vi "Table verify colomn.vi"(0 "PDF Report":T21(xcontrol), 5 "numColumns":i32, 9 "columnWidth":sgl[](array[numeric]), 11 "error in (no error)":errorcluster, 12 "Pages dimensions":T1={"Start at page"=-1, "Orientation"=enum."Portrait", "widht"=612.0, "height"=792.0, "Margin left"=72.0, "Margin right"=72.0, "Margin top"=72.0, "Margin bottom"=72.0}) -> (4 "PDF Report duplicate":T21(xcontrol), 6 "numColumns duplicate":i32, 10 "columnWidth (points)":sgl[](array[numeric]), 15 "error out":errorcluster)   [LabVIEW 2013]
doc: "Version 1.0\nDeveloped by Jean-Marc Simard\nCopyright © 2010, Exaprom Inc.\nAll rights reserved.\nLicense: BSD\n\nWith iTextSharp 4.1.6 (http://itextsharp.sourceforge.net)\nunder Mozilla Public License Version 1.1\n(http://www.mozilla.org/MPL/MPL-1.1.html)"
uses:
  Controls/PDF Report Xcontrol/PDF Report.xctl
  Controls/Page dimensions.ctl
  Controls/Page Orientation.ctl
  Controls/Unit.ctl
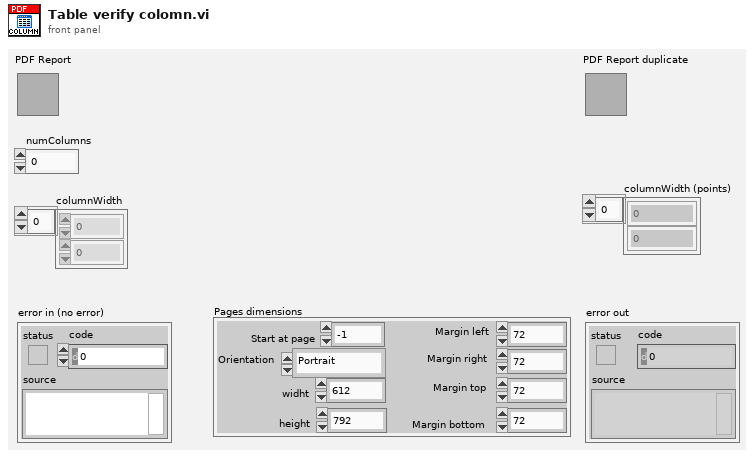
[diagram p1: front panel]
types:
  T1 = typedef "Page dimensions.ctl" = cluster{"Start at page":i32, "Orientation":T2, "widht":sgl, "height":sgl, "Margin left":sgl, "Margin right":sgl, "Margin top":sgl, "Margin bottom":sgl}
  T2 = typedef "Page Orientation.ctl" = enum16{"Portrait", "Landscape"}
  T3 = typedef "Font cluster.ctl" = cluster{"Name":string, "Size":T4, "Color":T5, "Style":cluster{"Bold":bool, "Italic":bool, "Underline":bool, "Strikeout":bool}}
  T4 = typedef "Font size.ctl" = sgl
  T5 = typedef "Font color.ctl" = u32
  T6 = typedef "Unit.ctl" = enum16{"inch", "mm"}
  T7 = typedef "Paragraphe cluster.ctl" = cluster{" Aligment":T8, "Line spacing":T9}
  T8 = typedef "Texte alignement.ctl" = enum16{"Select", "CENTER", "JUSTIFY", "LEFT", "RIGHT"}
  T9 = typedef "Line spacing.ctl" = enum16{"Select", "1.0", "1.5", "2.0"}
  T10 = typedef "Image or Table Caption.ctl" = cluster{"Caption":string, "Separator":string, "Position":enum16{"Above", "Below"}}
  T11 = typedef "Header Footer [ ].ctl" = T12[]
  T12 = typedef "Header Footer cluster.ctl" = cluster{"Start page":i32, "Type":T13, "Alignment":T14, "Vertical Alignement":T15, "Image (%)":sgl, "Page #":T16, "Text":string, "Path":string, "Font":T3, "Font refnum":refnum<k24>, "Line":cluster{"Line":T17, "Thickness (points)":sgl, "Colour":T5}}
  T13 = typedef "Header Footer Type.ctl" = enum16{"Select", "Text", "Text + hyperlink", "Page number", "Image", "Image + hyperlink"}
  T14 = typedef "Header footer horiz alignment.ctl" = enum16{"Left", "Center", "Right"}
  T15 = typedef "Cell Vertical alignment.ctl" = enum16{"TOP", "MIDDLE", "BOTTOM"}
  T16 = typedef "Page number.ctl" = cluster{"Text 1":string, "Text 2":string, "Text 3":string}
  T17 = typedef "Header Footer Line.ctl" = enum16{"No line", "Horizontal line"}
  T18 = typedef "Watermark cluster2.ctl" = cluster{"Show? (F)":bool, "Type":enum16{"Image", "Text"}, "Opacity (%)":sgl, "Rotate(°)":sgl, "Position":cluster{"Position":T19, "X":sgl, "Y":sgl}, "Image path":path, "Scaled(%)":sgl, "Image refnum":refnum<k24>, "Text":string, "Font":cluster{"Name":string, "Size":T4, "Color":T5}, "Font refnum":refnum<k24>, "Alignment":T14, "Automatic":bool}
  T19 = typedef "Watermark Position.ctl" = enum16{"Absolute", "Center (page)", "Center (text section)"}
  T20 = typedef "System Fonts.ctl" = cluster{"Font name [ ]":string[], "Font and file names [ ]":cluster{"Font name":string, "File name":string}[]}
  T21 = cluster{"Document":refnum<k24>, "Writer":refnum<k24>, "Default Font":refnum<k24>, "Default Font cluster":T3, "Path":path, "Unit (default = mm)":T6, "Paragraphe cluster":T7, "Pages dimensions [ ]":T1[], "Captions":cluster{"Image":T10, "Image counter":u16, "Table":T10, "Table counter":u16, "Font":T3}, "Header":T11, "Footer":T11, "Watermark ":T18, "Actual VI name":string, "System Fonts":T20}
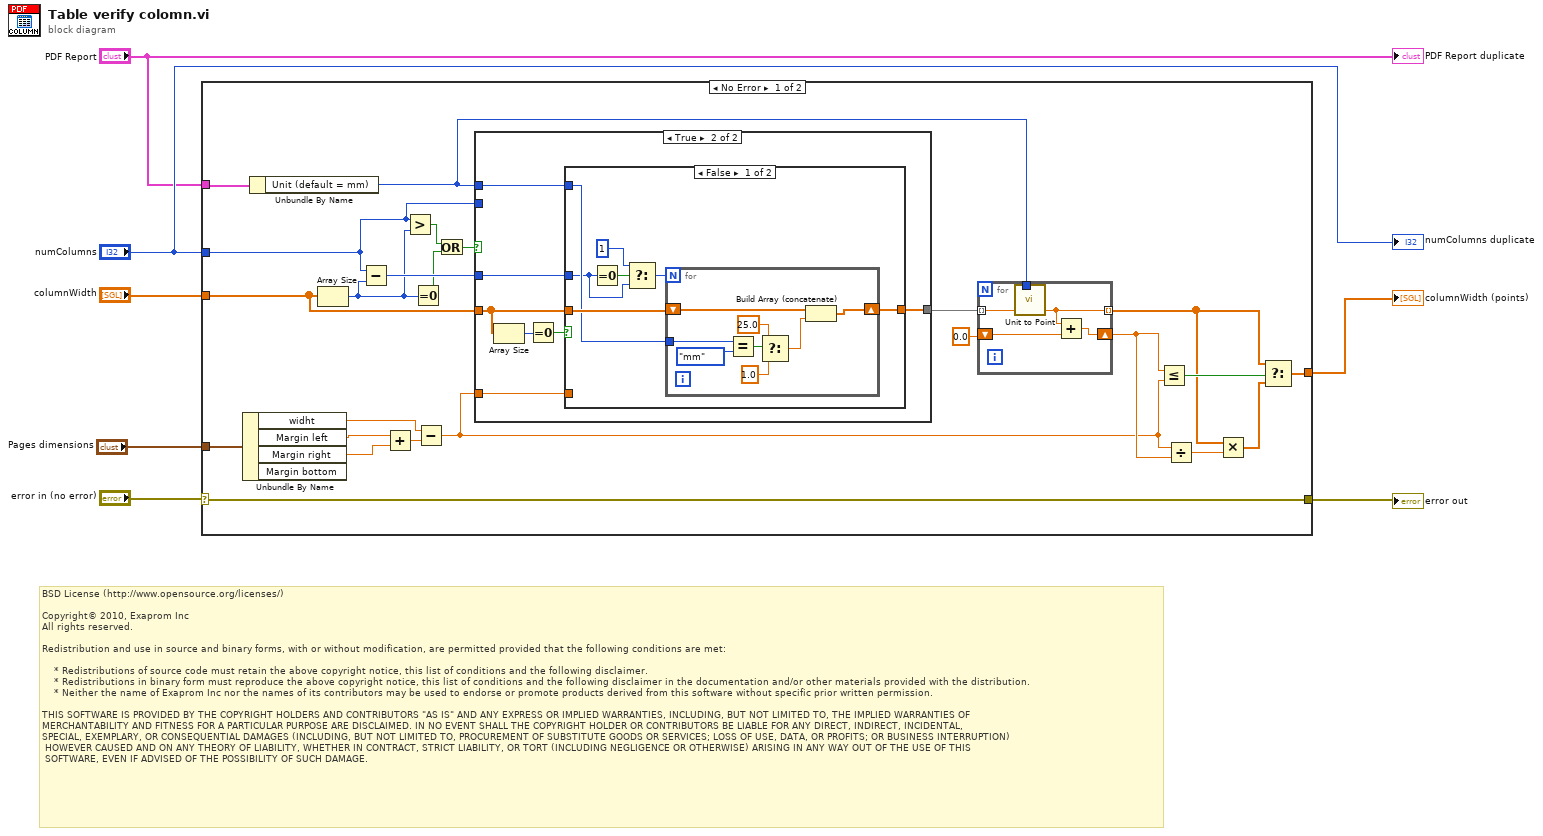
[diagram p0: block diagram]
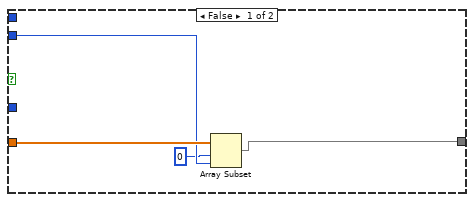
[diagram p2: hidden frame]
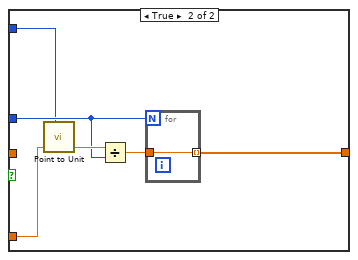
[diagram p3: hidden frame]
diagram:
  # "BSD License (http://www.opensource.org/licenses/)\n\nCopyright© 2010, Exaprom Inc\nAll rights reserved.\n\nRedistribution and use in source and binary forms, with or without modification, are permitted provided that the following conditions are met:\n\n    * Redistributions of source code must retain the above copyright notice, this list of conditions and the following disclaimer.\n    * Redistributions in binary form must reproduce the above copyright notice, this list of conditions and the following disclaimer in the documentation and/or other materials provided with the distribution.\n    * Neither the name of Exaprom Inc nor the names of its contributors may be used to endorse or promote products derived from this software without specific prior written permission.\n\nTHIS SOFTWARE IS PROVIDED BY THE COPYRIGHT HOLDERS AND CONTRIBUTORS \"AS IS\" AND ANY EXPRESS OR IMPLIED WARRANTIES, INCLUDING, BUT NOT LIMITED TO, THE IMPLIED WARRANTIES OF \nMERCHANTABILITY AND FITNESS FOR A PARTICULAR PURPOSE ARE DISCLAIMED. IN NO EVENT SHALL THE COPYRIGHT HOLDER OR CONTRIBUTORS BE LIABLE FOR ANY DIRECT, INDIRECT, INCIDENTAL,\nSPECIAL, EXEMPLARY, OR CONSEQUENTIAL DAMAGES (INCLUDING, BUT NOT LIMITED TO, PROCUREMENT OF SUBSTITUTE GOODS OR SERVICES; LOSS OF USE, DATA, OR PROFITS; OR BUSINESS INTERRUPTION)\n HOWEVER CAUSED AND ON ANY THEORY OF LIABILITY, WHETHER IN CONTRACT, STRICT LIABILITY, OR TORT (INCLUDING NEGLIGENCE OR OTHERWISE) ARISING IN ANY WAY OUT OF THE USE OF THIS\n SOFTWARE, EVEN IF ADVISED OF THE POSSIBILITY OF SUCH DAMAGE."
  n1 = case shown="No Error" "error in (no error)" {
    selector: "error in (no error)" -> [w17 w71]
    tunnel: "columnWidth" -> [w15 w70]
    tunnel: "numColumns" -> [w22 _]
    tunnel: "Pages dimensions" -> [w16 _]
    tunnel: [w18 w70] -> w6
    tunnel: [w17 w71] -> w4
    tunnel: "PDF Report" -> [w13 _]
    frame No Error {
      n2 = Unbundle By Name(w16) -> ("widht"=w30:sgl, "Margin left"=w28:sgl, "Margin right"=w29:sgl)  [unwired: 1 out]
      n3 = Unbundle By Name(w13) -> ("Unit (default = mm)"=w12:T6)
      n4 = Array Size(array=w15) -> (size(s)=w8:i32)
      n5 = Subtract(x=w22, y=w8) -> (x-y=w23:i32)
      n6 = Add(x=w28, y=w29) -> (x+y=w31:sgl)
      n7 = Greater?(x=w22, y=w8) -> (0:w10:bool)
      n8 = Equal To 0?(x=w8) -> (x = 0?=w9:bool)
      n9 = Subtract(x=w30, y=w31) -> (x-y=w14:sgl)
      n10 = Or(x=w10, y=w9) -> (x .or. y?=w11:bool)
      n11 = case shown="True" w11 {
        tunnel: w15 -> [w35 w40]
        tunnel: w23 -> [_ w42]
        tunnel: w22 -> [w34 _]
        tunnel: [w32 w41] -> w21
        tunnel: w14 -> [_ w37]
        tunnel: w12 -> [_ w36]
        frame False {
          n12 = Array Subset(array=w35, index=0, length=w34) -> (w32:sgl[])
        }
        frame True {
          n13 = Array Size(array=w40) -> (size(s)=w39:i32)
          n14 = Equal To 0?(x=w39) -> (x = 0?=w38:bool)
          n15 = case shown="False" w38 {
            tunnel: w42 -> [w44 w60]
            tunnel: [w49 w63] -> w41
            tunnel: w40 -> [w48 _]
            tunnel: w37 -> [_ w62]
            tunnel: w36 -> [w47 w58]
            frame False {
              n16 = Equal To 0?(x=w44) -> (x = 0?=w46:bool)
              n17 = Select(t=1, s=w46, f=w44) -> (s? t:f=w45:i32)
              n18 = for {
                N: w45 -> [_]
                shift-right: [w56] -> w49
                shift-left: w48 -> [w57]
                tunnel: w47 -> [w55]
                n19 = Equal?(x=w55, y=Unit."mm") -> (x = y?=w53:bool)
                n20 = Select(t=sgl 25.0 ("mm"), s=w53, f=sgl 1.0 ("mm")) -> (s? t:f=w51:sgl)
                n21 = Build Array (concatenate)(w57, w51) -> (w56:sgl[])
              }
            }
            frame True {
              n22 = call "Point to Unit.vi"("X point"=w62, "Unit (default = mm)"=w58) -> ("X unit"=w61:sgl)  [unwired: 7 out]
              n23 = Divide(x=w61, y=w60) -> (x/y=w59:sgl)
              n24 = for {
                N: w60 -> [_]
                tunnel: [w64] -> w63 mode=indexing
                tunnel: w59 -> [w64]
              }
            }
          }
        }
      }
      n25 = for {
        tunnel: w21 -> [w69] mode=indexing
        tunnel: [w67] -> w19 mode=indexing
        shift-right: [w66] -> w24
        shift-left: sgl 0.0 ("WidthPercentage") -> [w68]
        tunnel: w12 -> [w65]
        n26 = call "Unit to Point.vi"("X unit"=w69, "Unit (default = mm)"=w65) -> ("X point"=w67:sgl)  [unwired: 7 out]
        n27 = Add(x=w67, y=w68) -> (x+y=w66:sgl)
      }
      n28 = Less Or Equal?(x=w24, y=w14) -> (x <= y?=w20:bool)
      n29 = Divide(x=w14, y=w24) -> (x/y=w26:sgl)
      n30 = Multiply(x=w19, y=w26) -> (x*y=w25:sgl[])
      n31 = Select(t=w19, s=w20, f=w25) -> (s? t:f=w18:sgl[])
    }
    frame Error {
    }
  }
  "columnWidth (points)" <- w6
  "error out" <- w4
  "PDF Report duplicate" <- "PDF Report"
  "numColumns duplicate" <- "numColumns"
